vi "Initialize DAQ (Onboard Clk).vi"(8 "error in (no error)":errorcluster, 10 "DAQ Settings":T2, 11 "DAQmx Resource":tag) -> (0 "error out":errorcluster, 3 "DAQmx Tasks":T1)   [LabVIEW 2025]
uses:
  <vilib>/DAQmx/write.llb/DAQmx Write (Digital Wfm 1Chan NSamp).vi
  <vilib>/Waveform/DWDTOps.llb/DWDT Append Digital Samples.vi
  <vilib>/Waveform/DWDTOps.llb/DWDT Digital Size.vi
  <vilib>/DAQmx/configure/timing.llb/DAQmx Timing (Sample Clock).vi
  <vilib>/Waveform/DWDTOps.llb/DWDT Uncompress Digital.vi
  <vilib>/DAQmx/miscellaneous.llb/DAQmx Fill In Error Info.vi
  <resource>/objmgr/daqmx.rc
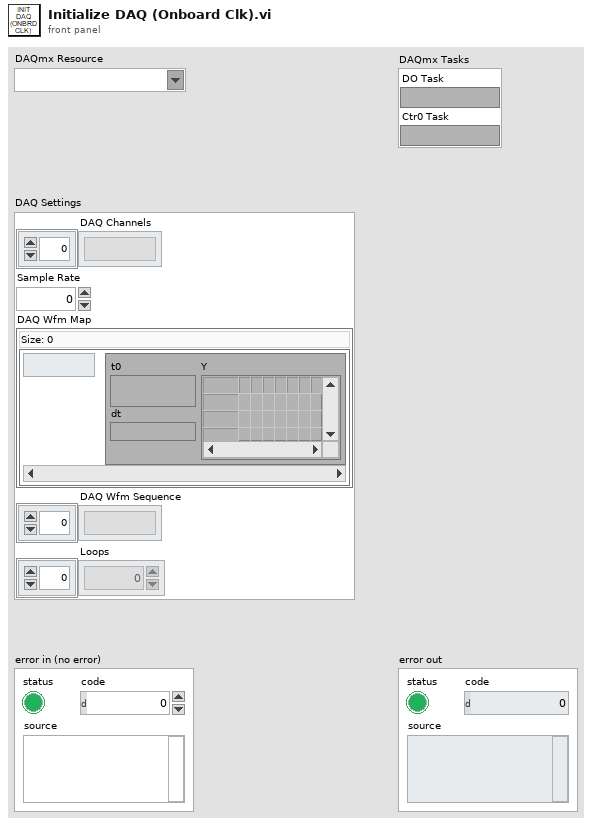
[diagram p1: front panel]
types:
  T1 = cluster{"DO Task":refnum<k21>, "Ctr0 Task":refnum<k21>}
  T2 = cluster{"DAQ Channels":string[], "Sample Rate":dbl, "DAQ Wfm Map":map{string, digitalwaveform}, "DAQ Wfm Sequence":string[], "Loops":i32[]}
  T3 = cluster{"task out":refnum<k21>, "Ctr0 Task":refnum<k21>}
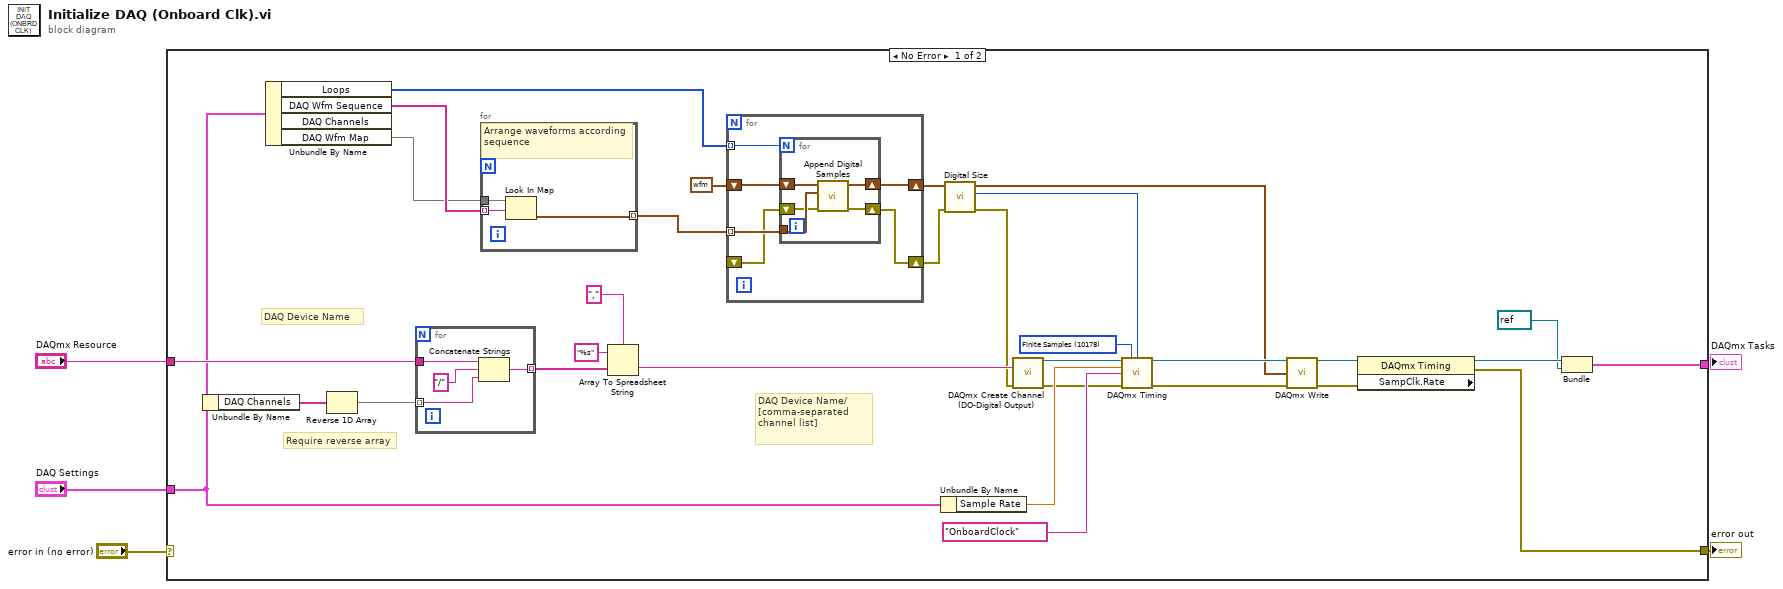
[diagram p0: block diagram]
diagram:
  n1 = case shown="No Error" "error in (no error)" {
    selector: "error in (no error)" -> [_ w54]
    tunnel: [w14 w54] -> w4
    tunnel: "DAQmx Resource" -> [w25 _]
    tunnel: "DAQ Settings" -> [w11 _]
    tunnel: [w19 _] -> _
    frame No Error {
      w6 = 10178 items=["Finite Samples"=10178, "Continuous Samples"=10123, "Hardware Timed Single Point"=12522] ("sample mode")
      # "Require reverse array"
      # "DAQ Device Name/[comma-separated channel list]"
      # "DAQ Device Name"
      n2 = Unbundle By Name(w11) -> ("DAQ Channels"=w34:string[])
      n3 = Unbundle By Name(w11) -> ("Loops"=w18:i32[], "DAQ Wfm Sequence"=w35:string[], "DAQ Wfm Map"=w29:map{string, digitalwaveform})  [unwired: 1 out]
      n4 = Reverse 1D Array(array=w34) -> (reversed array=w15:string[])
      n5 = for {
        tunnel: w25 -> [w53]
        tunnel: w15 -> [w51] mode=indexing
        tunnel: [w50] -> w33 mode=indexing
        n6 = Concatenate Strings(w53, "/", w51) -> (w50:string)
      }
      n7 = for {
        tunnel: w35 -> [w49] mode=indexing
        tunnel: w29 -> [w48]
        tunnel: [w47] -> w28 mode=indexing
        # "Arrange waveforms according sequence"
        n8 = Look In Map(map=w48, key=w49) -> (value=w47:digitalwaveform)  [unwired: 1 in, 1 out]
      }
      n9 = Array To Spreadsheet String(delimiter (Tab)=",", array=w33, 3:"%s" ("format string")) -> (spreadsheet string=w30:string)
      n10 = for {
        shift-right: [w40] -> w24
        shift-left: digitalwaveform {"t0"=timestamp(0 s since 1904-01-01), "dt"=0.0, "Y"={"transitions"=[], "data"=[]}} ("digital waveform out") -> [w41]
        tunnel: w28 -> [w39] mode=indexing
        shift-right: [w37] -> w22
        shift-left: _ -> [w38]
        tunnel: w18 -> [w36] mode=indexing
        n11 = for {
          N: w36 -> [_]
          tunnel: w39 -> [w44]
          shift-right: [w45] -> w40
          shift-left: w41 -> [w46]
          shift-right: [w42] -> w37
          shift-left: w38 -> [w43]
          n12 = call-poly <vilib>:"Append Digital Samples.vi"("error in (no error)"=w43, "digital waveform B"=w44, "digital waveform A"=w46) -> ("error out"=w42:errorcluster, "digital waveform out"=w45:digitalwaveform)  [unwired: 7 in]
        }
      }
      n13 = Unbundle By Name(w11) -> ("Sample Rate"=w10:dbl)
      n14 = call-poly <vilib>:"Digital Size.vi"("error in (no error)"=w22, "digital waveform in"=w24) -> ("error out"=w21:errorcluster, "number of samples"=w23:i32, "digital waveform out"=w16:digitalwaveform)  [unwired: 6 in, 1 out]
      n15 = call <vilib>:"DAQmx Create Channel (DO-Digital Output).vi"("lines"=w30, "error in"=w21) -> ("task out"=w7:refnum<k21>, "error out"=w8:errorcluster)  [unwired: 12 in]
      n16 = call-poly <vilib>:"DAQmx Timing.vi"("task/channels in"=w7, "sample mode"=w6, "samples per channel"=w23, "rate"=w10, "source"=tag "OnboardClock", "error in"=w8) -> ("task out"=w26:refnum<k21>, "error out"=w20:errorcluster)  [unwired: 8 in]
      n17 = call-poly <vilib>:"DAQmx Write.vi"("task/channels in"=w26, "data"=w16, "error in"=w20) -> ("task out"=w13:refnum<k21>, "error out"=w27:errorcluster)  [unwired: 10 in, 1 out]
      n18 = property class="DAQmx Timing" props=["SampClk.Rate"](reference=w13, error in=w27) -> (reference out=w12:refnum<k21>, error out=w14:errorcluster)  [unwired: 1 out]
      n19 = Bundle("task out"=w12, "Ctr0 Task"=refnum<k21> refnum) -> (w19:T3)  [unwired: 1 in]
    }
    frame Error {
    }
  }
  "error out" <- w4
